vi "UpdateSymbolInDir.vi"(8 "error in":errorcluster, 10 "Name":string="LabVIEW 2014", 11 "Path":path=path "D:/") -> (0 "error out":errorcluster, 3 "Path (dup)":path=path "D:/")   [LabVIEW 2014]
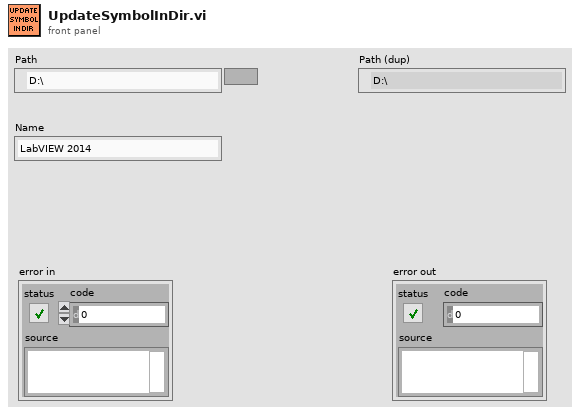
[diagram p1: front panel]
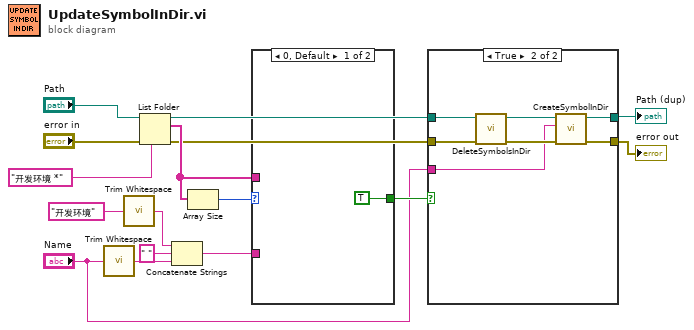
[diagram p0: block diagram]
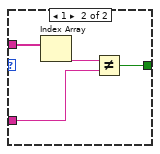
[diagram p3: hidden frame]
diagram:
  n1 = call <vilib>:"Trim Whitespace.vi"("string"="Name") -> ("trimmed string"=w10:string)  [unwired: 1 in]
  n2 = call <vilib>:"Trim Whitespace.vi"("string"="开发环境" ("Name")) -> ("trimmed string"=w9:string)  [unwired: 1 in]
  n3 = List Folder(path="Path", pattern="开发环境 *", error in="error in") -> (path out=w4:path, filenames=w7:string[], error out=w5:errorcluster)  [unwired: 1 in, 1 out]
  n4 = Concatenate Strings(w9, " " ("string"), w10) -> (w8:string)
  n5 = Array Size(array=w7) -> (size(s)=w13:i32)
  n6 = case shown="0, Default" w13 {
    tunnel: w8 -> [_ w19]
    tunnel: w7 -> [_ w21]
    tunnel: [TRUE w18] -> w6
    frame 0, Default {
    }
    frame 1 {
      n7 = Index Array(array=w21) -> (element=w20:string)  [unwired: 1 in]
      n8 = Not Equal?(x=w20, y=w19) -> (x != y?=w18:bool)
    }
  }
  n9 = case shown="True" w6 {
    tunnel: w5 -> [w22 w28]
    tunnel: w4 -> [w23 w27]
    tunnel: "Name" -> [_ w26]
    tunnel: [w23 w25] -> w2
    tunnel: [w22 w24] -> w1
    frame False {
    }
    frame True {
      n10 = call "DeleteSymbolsInDir.vi"("error in (no error)"=w28, "dup path"=w27) -> ("error in (no error) (dup)"=w29:errorcluster, "dup path (dup)"=w30:path)  [unwired: 8 in]
      n11 = call "CreateSymbolInDir.vi"("error in"=w29, "Name"=w26, "Path"=w30) -> ("error out"=w24:errorcluster, "Path (dup)"=w25:path)  [unwired: 7 in]
    }
  }
  "error out" <- w1
  "Path (dup)" <- w2
